vi "control_ttl_protocol_from_textfile.vi"(9 "Input \nparameters":T2={"Frame rate (ms)"=2000, "Worm strain"="N2", "Time t"=0, "State"=enum."Initialize measurement", "Time elapsed"=0.0, "Max_num_runs"=100000, "#TTL"=0, "Time of start TTL"=100000, "ImSub Value"=0, "Time of last TTL"=0, "Number of Columns"=2, "Number of Rows"=2, "# AdjacentTTL"=0, "Sleep deprivation status"="", "Sleep detection"=FALSE, "# Sleep detections"=0, "Time of first sleep detection"=0, "Time max # adjacent TTL"=0, "Image t-1"=[], "Image t"=[]} {"Number of Rows" items=["1"=1, "2"=2, "3"=3, "4"=4]; "Number of Columns" items=["1"=1, "2"=2, "3"=3, "4"=4]}) -> (1 "Output \nparameters":T2={"Frame rate (ms)"=2000, "Worm strain"="N2", "Time t"=0, "State"=enum."Initialize measurement", "Time elapsed"=0.0, "Max_num_runs"=100000, "#TTL"=0, "Time of start TTL"=100000, "ImSub Value"=0, "Time of last TTL"=0, "Number of Columns"=2, "Number of Rows"=2, "# AdjacentTTL"=0, "Sleep deprivation status"="", "Sleep detection"=FALSE, "# Sleep detections"=0, "Time of first sleep detection"=0, "Time max # adjacent TTL"=0, "Image t-1"=[], "Image t"=[]} {"Number of Rows" items=["1"=1, "2"=2, "3"=3, "4"=4]; "Number of Columns" items=["1"=1, "2"=2, "3"=3, "4"=4]})   [LabVIEW 2011]
uses:
  state.ctl
  <vilib>/Utility/file.llb/Read From Spreadsheet File (DBL).vi
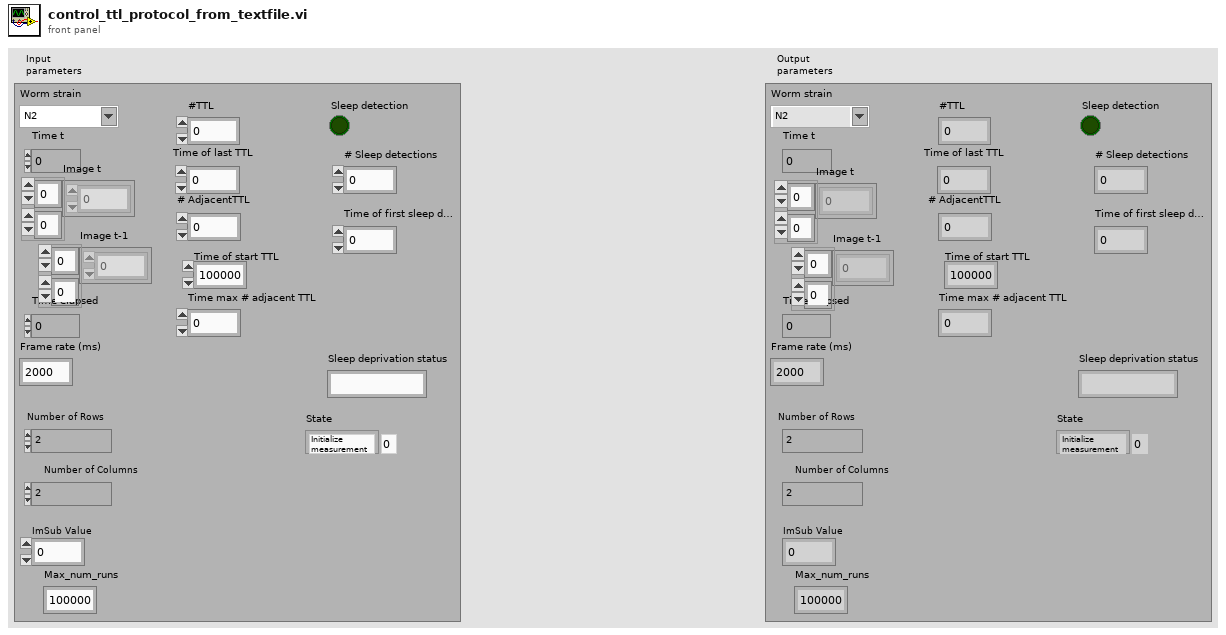
[diagram p1: front panel]
types:
  T1 = typedef "state.ctl" = enum16{"Initialize measurement", "Image acquisition", "Image processing", "Sleep detection", "Control TTL protocol ", "Sleep deprivation", "Update image & exit condition", "Wait "}
  T2 = cluster{"Frame rate (ms)":u32, "Worm strain":string, "Time t":i32, "State":T1, "Time elapsed":dbl, "Max_num_runs":i32, "#TTL":i32, "Time of start TTL":i32, "ImSub Value":i32, "Time of last TTL":i32, "Number of Columns":u32, "Number of Rows":u32, "# AdjacentTTL":i32, "Sleep deprivation status":string, "Sleep detection":bool, "# Sleep detections":i32, "Time of first sleep detection":i32, "Time max # adjacent TTL":i32, "Image t-1":i32[][], "Image t":i32[][]}
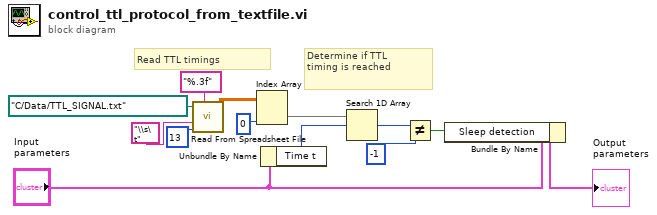
[diagram p0: block diagram]
diagram:
  # "Determine if TTL \ntiming is reached"
  # "Read TTL timings"
  n1 = call-poly <vilib>:"Read From Spreadsheet File.vi"("delimiter (\\t)"="\\s\t" ("delimiter (\\t)"), "format (%.3f)"="%.3f", "max characters/row  (no limit:0)"=13, "file path (dialog if empty)"=path "C:/Data/TTL_SIGNAL.txt") -> ("all rows"=w8:dbl[][])  [unwired: 3 in, 4 out]
  n2 = Index Array(array=w8, index (col)=0 ("Deaktivierter Index (Spalte)")) -> (element=w4:dbl[])  [unwired: 1 in]
  n3 = Unbundle By Name("Input \nparameters") -> ("Time t"=w5:i32)
  n4 = Search 1D Array(1D array=w4, element=w5) -> (index of element=w7:i32)  [unwired: 1 in]
  n5 = Not Equal?(x=w7, y=-1) -> (x != y?=w3:bool)
  n6 = Bundle By Name(cluster="Input \nparameters", "Sleep detection"=w3) -> (→"Output \nparameters":T2)
